vi "Rename Project.vi"(8 "error in (no error)":errorcluster, 11 "ProjectItem in":refnum<class "ProjectItem.lvclass">) -> (0 "error out":errorcluster, 3 "ProjectItem out":refnum<class "ProjectItem.lvclass">)   [LabVIEW 2019, in "ProjectItem.lvclass"]
uses:
  ProjectItem.lvclass
  ProjectItem.lvclass/ProjectItem.ctl
  <vilib>/regexp/Match Regular Expression.xnode
panel:
  out "Project Name":string
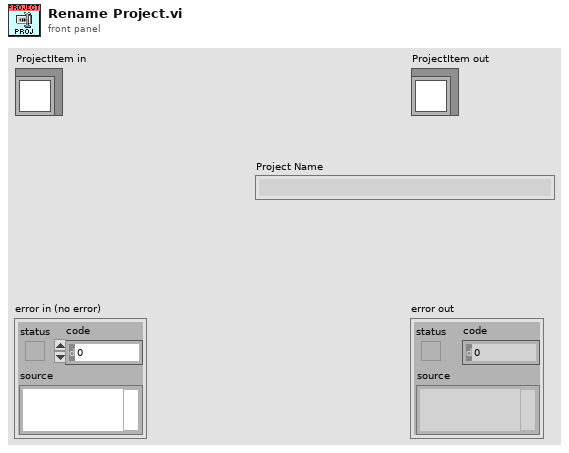
[diagram p1: front panel]
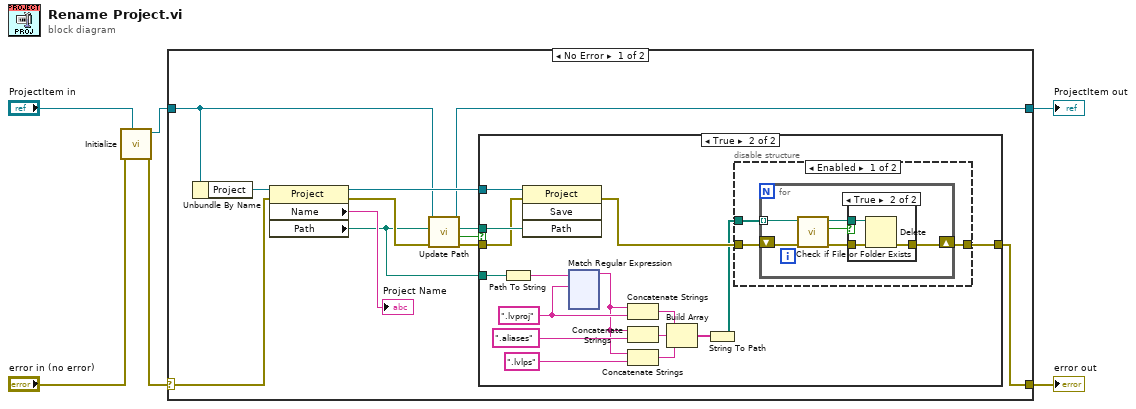
[diagram p0: block diagram]
diagram:
  n1 = call "Initialize.vi"("ProjectItem"="ProjectItem in", "error in (no error)"="error in (no error)") -> ("error out"=w1:errorcluster, "ProjectItem out"=w3:refnum<class "ProjectItem.lvclass">)  [unwired: 8 in]
  n2 = case shown="No Error" w1 {
    selector: w1 -> [w15 w165]
    tunnel: [w7 w165] -> w6
    tunnel: [w14 w164] -> w5
    tunnel: w3 -> [w12 w164]
    frame No Error {
      n3 = Unbundle By Name(w12) -> ("Project"=w16:refnum<vi>)
      n4 = property class="Project"(reference=w16, error in=w15) -> (reference out=w17:refnum<vi>, error out=w11:errorcluster, "Name"=→"Project Name":string, "Path"=w8:path)
      n5 = call "Update Path.vi"("error in (no error)"=w11, "Path in"=w8, "Rename in"=w12) -> ("error out"=w10:errorcluster, "New Path?"=w9:bool, "Path out"=w18:path, "Rename out"=w14:refnum<class "ProjectItem.lvclass">)  [unwired: 5 in]
      n6 = case shown="True" w9 {
        tunnel: w18 -> [_ w35]
        tunnel: w17 -> [_ w34]
        tunnel: [w19 w32] -> w7
        tunnel: w10 -> [w19 w33]
        tunnel: w8 -> [_ w30]
        frame False {
        }
        frame True {
          w26 = ".lvproj" ("format string")
          n7 = Path To String(path=w30) -> (string=w29:string)
          n8 = invoke class="Project" method="Save"(reference=w34, error in=w33, "Path"=w35) -> (error out=w31:errorcluster)  [unwired: 1 in, 3 out]
          n9 = xnode "Match Regular Expression"("input string"=w29, "regular expression"=w26) -> ("before match"=w20:string)  [unwired: 4 in, 4 out]
          n10 = Concatenate Strings(w20, w26) -> (w22:string)
          n11 = Concatenate Strings(w20, ".aliases" ("string")) -> (w25:string)
          n12 = Concatenate Strings(w20, ".lvlps" ("string")) -> (w23:string)
          n13 = Build Array(w22, w25, w23) -> (w24:string[])
          n14 = String To Path(string=w24) -> (path=w21:path[])
          n15 = disable-structure shown="Enabled" {
            disable-tunnel: w31 -> [w152 w163]
            disable-tunnel: [w151 w163] -> w32
            disable-tunnel: w21 -> [w150 _]
            frame Enabled {
              n16 = for {
                tunnel: w150 -> [w157] mode=indexing
                shift-right: [w158] -> w151
                shift-left: w152 -> [w156]
                n17 = call <vilib>:"Check if File or Folder Exists.vi"("error in (no error)"=w156, "path"=w157) -> ("error out"=w155:errorcluster, "file or folder exists?"=w154:bool, "dup path"=w153:path)  [unwired: 7 in]
                n18 = case shown="True" w154 {
                  tunnel: w155 -> [w159 w162]
                  tunnel: [w159 w161] -> w158
                  tunnel: w153 -> [_ w160]
                  frame False {
                  }
                  frame True {
                    n19 = Delete(path (use dialog)=w160, error in=w162) -> (error out=w161:errorcluster)  [unwired: 3 in, 2 out]
                  }
                }
              }
            }
            frame Disabled {
            }
          }
        }
      }
    }
    frame Error {
    }
  }
  "error out" <- w6
  "ProjectItem out" <- w5
